vi "check_signal_chopper_state.vi"(7 "parity?":bool, 8 "Enum":enum16{"mod2", "mod4"}(ring)=enum."mod4", 9 "PD in":dbl[](array[numeric]), 10 "chopper":bool[](array[boolean]), 11 "data":dbl[][](array[numeric])) -> (1 "PD out":dbl[](array[numeric]), 2 "chopper out":bool[](array[boolean]), 3 "data out":dbl[][](array[numeric]))   [LabVIEW 2019]
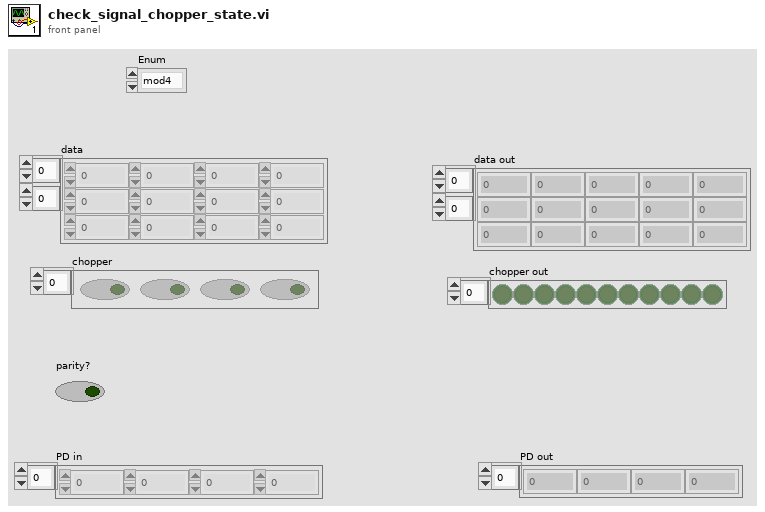
[diagram p1: front panel]
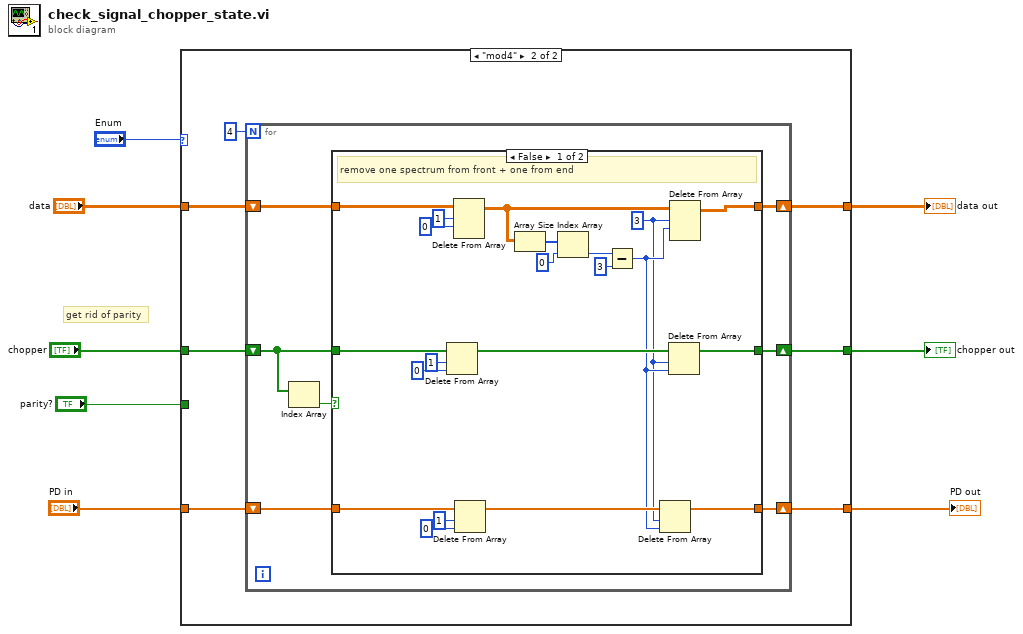
[diagram p0: block diagram]
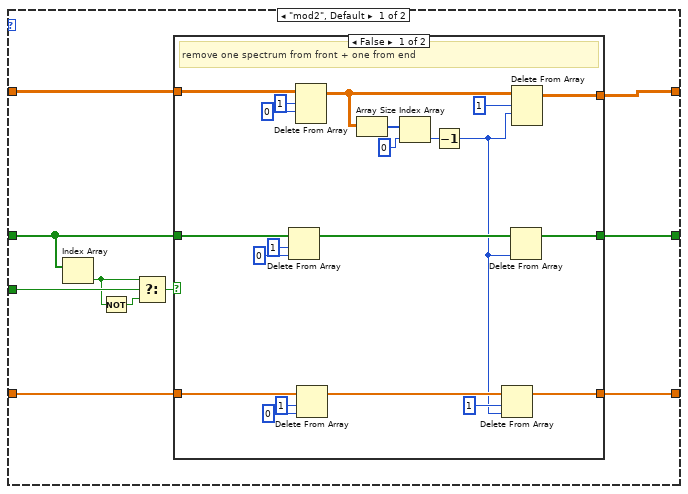
[diagram p2: hidden frame]
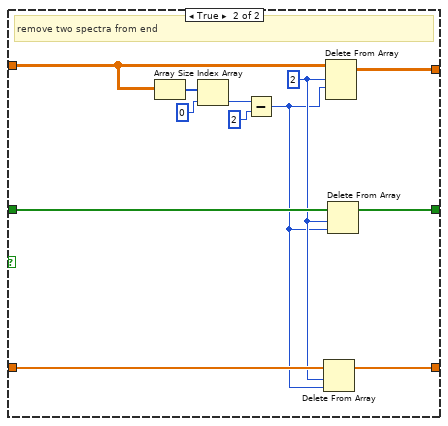
[diagram p3: hidden frame]
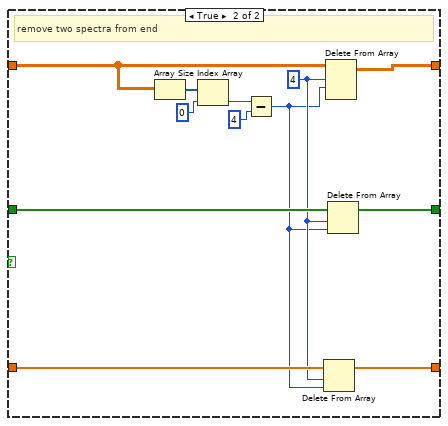
[diagram p4: hidden frame]
diagram:
  # "get rid of parity"
  n1 = case shown="\"mod4\"" "Enum" {
    tunnel: [w18 w55] -> w8
    tunnel: [w17 w54] -> w7
    tunnel: "parity?" -> [w16 _]
    tunnel: "chopper" -> [w14 w56]
    tunnel: "data" -> [w11 w58]
    tunnel: "PD in" -> [w10 w57]
    tunnel: [w9 w53] -> w2
    frame "mod2", Default {
      n2 = Index Array(array=w14) -> (element=w13:bool)  [unwired: 1 in]
      n3 = Not(x=w13) -> (.not. x?=w12:bool)
      n4 = Select(t=w13, s=w16, f=w12) -> (s? t:f=w15:bool)
      n5 = case shown="False" w15 {
        tunnel: w11 -> [w33 w48]
        tunnel: [w37 w49] -> w18
        tunnel: w14 -> [w29 w45]
        tunnel: [w26 w44] -> w17
        tunnel: w10 -> [w23 w43]
        tunnel: [w19 w42] -> w9
        frame False {
          # "remove one spectrum from front + one from end"
          n6 = Delete From Array(array=w29, length=1, index=0 ("index (row)")) -> (array with subset deleted=w28:bool[])  [unwired: 1 out]
          n7 = Delete From Array(array=w33, length=1, index (row)=0) -> (array with subset deleted=w32:dbl[][])  [unwired: 1 in, 1 out]
          n8 = Delete From Array(array=w23, length=1, index=0 ("index (row)")) -> (array with subset deleted=w22:dbl[])  [unwired: 1 out]
          n9 = Array Size(array=w32) -> (size(s)=w36:i32[])
          n10 = Index Array(array=w36, index=0) -> (element=w34:i32)
          n11 = Decrement(x=w34) -> (x-1=w20:i32)
          n12 = Delete From Array(array=w22, length=1, index=w20) -> (array with subset deleted=w19:dbl[])  [unwired: 1 out]
          n13 = Delete From Array(array=w28, index=w20) -> (array with subset deleted=w26:bool[])  [unwired: 1 in, 1 out]
          n14 = Delete From Array(array=w32, length=1, index (row)=w20) -> (array with subset deleted=w37:dbl[][])  [unwired: 1 in, 1 out]
        }
        frame True {
          w41 = 2 ("length")
          # "remove two spectra from end"
          n15 = Array Size(array=w48) -> (size(s)=w51:i32[])
          n16 = Index Array(array=w51, index=0) -> (element=w47:i32)
          n17 = Subtract(x=w47, y=2) -> (x-y=w40:i32)
          n18 = Delete From Array(array=w43, length=w41, index=w40) -> (array with subset deleted=w42:dbl[])  [unwired: 1 out]
          n19 = Delete From Array(array=w48, length=w41, index (row)=w40) -> (array with subset deleted=w49:dbl[][])  [unwired: 1 in, 1 out]
          n20 = Delete From Array(array=w45, length=w41, index=w40) -> (array with subset deleted=w44:bool[])  [unwired: 1 out]
        }
      }
    }
    frame "mod4" {
      n21 = for {
        N: 4 -> [_]
        shift-right: [w61] -> w55
        shift-left: w58 -> [w65]
        shift-right: [w60] -> w54
        shift-left: w56 -> [w63]
        shift-right: [w59] -> w53
        shift-left: w57 -> [w64]
        n22 = Index Array(array=w63) -> (element=w62:bool)  [unwired: 1 in]
        n23 = case shown="False" w62 {
          tunnel: w65 -> [w81 w95]
          tunnel: [w84 w96] -> w61
          tunnel: w63 -> [w77 w92]
          tunnel: [w75 w91] -> w60
          tunnel: w64 -> [w72 w90]
          tunnel: [w70 w89] -> w59
          frame False {
            w66 = 3 ("length")
            # "remove one spectrum from front + one from end"
            n24 = Delete From Array(array=w77, length=1, index=0 ("index (row)")) -> (array with subset deleted=w76:bool[])  [unwired: 1 out]
            n25 = Delete From Array(array=w81, length=1, index (row)=0) -> (array with subset deleted=w80:dbl[][])  [unwired: 1 in, 1 out]
            n26 = Delete From Array(array=w72, length=1, index=0 ("index (row)")) -> (array with subset deleted=w71:dbl[])  [unwired: 1 out]
            n27 = Array Size(array=w80) -> (size(s)=w83:i32[])
            n28 = Index Array(array=w83, index=0) -> (element=w69:i32)
            n29 = Subtract(x=w69, y=3) -> (x-y=w68:i32)
            n30 = Delete From Array(array=w71, length=w66, index=w68) -> (array with subset deleted=w70:dbl[])  [unwired: 1 out]
            n31 = Delete From Array(array=w76, length=w66, index=w68) -> (array with subset deleted=w75:bool[])  [unwired: 1 out]
            n32 = Delete From Array(array=w80, length=w66, index (row)=w68) -> (array with subset deleted=w84:dbl[][])  [unwired: 1 in, 1 out]
          }
          frame True {
            w88 = 4 ("length")
            # "remove two spectra from end"
            n33 = Array Size(array=w95) -> (size(s)=w98:i32[])
            n34 = Index Array(array=w98, index=0) -> (element=w94:i32)
            n35 = Subtract(x=w94, y=4) -> (x-y=w87:i32)
            n36 = Delete From Array(array=w90, length=w88, index=w87) -> (array with subset deleted=w89:dbl[])  [unwired: 1 out]
            n37 = Delete From Array(array=w95, length=w88, index (row)=w87) -> (array with subset deleted=w96:dbl[][])  [unwired: 1 in, 1 out]
            n38 = Delete From Array(array=w92, length=w88, index=w87) -> (array with subset deleted=w91:bool[])  [unwired: 1 out]
          }
        }
      }
    }
  }
  "data out" <- w8
  "chopper out" <- w7
  "PD out" <- w2
